vi "[RT]CTRL_PumpValve.vi"(11 "target-volume":dbl) -> (2 "volume reached":bool, 3 "pressure reached":bool)   [LabVIEW 2018]
uses:
  [GlobVar]SensorState.vi
  [GlobVar]Param.vi
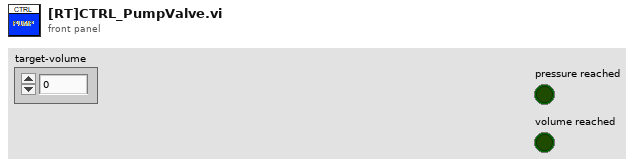
[diagram p1: front panel]
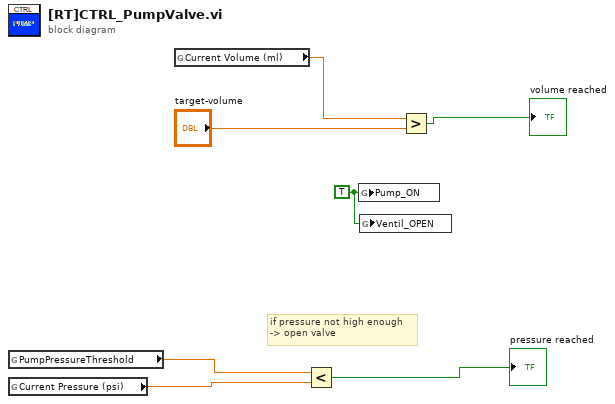
[diagram p0: block diagram]
diagram:
  w2 = TRUE ("Pump_ON")
  # "if pressure not high enough\n-> open valve"
  n1 = global read "[GlobVar]Param.vi" "PumpPressureThreshold"() -> (w7:dbl)
  n2 = global read "[GlobVar]SensorState.vi" "Current Pressure (psi)"() -> (w3:dbl)
  n3 = global read "[GlobVar]SensorState.vi" "Current Volume (ml)"() -> (w5:dbl)
  n4 = Less?(x=w7, y=w3) -> (x < y?=→"pressure reached":bool)
  n5 = global write "[GlobVar]SensorState.vi" "Pump_ON"(w2) -> ()
  n6 = global write "[GlobVar]SensorState.vi" "Ventil_OPEN"(w2) -> ()
  n7 = Greater?(x=w5, y="target-volume") -> (0:→"volume reached":bool)
